vi "Main.vi"() -> ()   [LabVIEW 2019]
uses:
  <vilib>/NI/Current Value Table/Type Defs/File Format.ctl
  <vilib>/NI/Current Value Table/Type Defs/Single Tag.ctl
  <vilib>/NI/Current Value Table/Type Defs/Data Types.ctl
  <vilib>/NI/Current Value Table/Type Defs/Tag Grouping set.ctl
  QDMH support files/QDMH Poly VIs/QDMH POLY Enqueue String.vi
  <vilib>/NI/Current Value Table/Current Value Table.lvlib
panel:
  in  "Ordem de serviço 2":string
  in  "Temperatura 2":dbl
  in  "Temperatura 1":dbl
  in  "Ferramentas":string
  in  "Queue Name":string="Main-PoC"
  out "error out":errorcluster
  in  "error in (no error)":errorcluster
  out "Message Display":string
  in  "Cancel":bool
  in  "OK":bool
  in  "Ordem de serviço":string
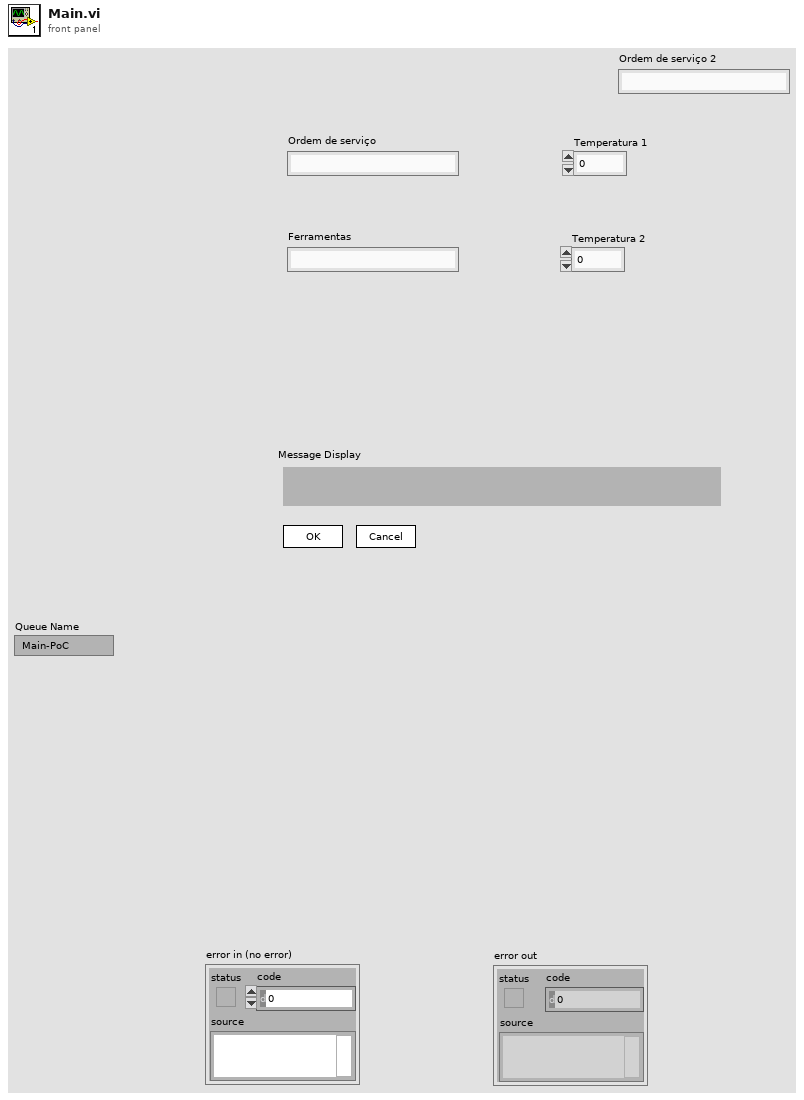
[diagram p1: front panel]
types:
  T1 = cluster{"Barcode to be sent":string, "Read code on next":bool, "New data?":bool, "SO code":cluster{"Current Barcode":string, "Ready to send?":bool, "New data to be polled?":bool}, "Tool code":cluster{"Current Barcode":string, "Ready to send?":bool, "New data to be polled?":bool}, "Polled Data to be sent":string}
  T2 = typedef "Current Value Table.lvlib/File Format.ctl" = cluster{"Tags":T3[], "Group Listings":T5[]}
  T3 = typedef "Current Value Table.lvlib/Single Tag.ctl" = cluster{"Data Type":T4, "Name":string, "Value":string, "Description":string}
  T4 = typedef "Current Value Table.lvlib/Data Types.ctl" = enum16{"Double", "Single", "I64", "I32", "I16", "I8", "U64", "U32", "U16", "U8", "String", "Boolean", "Array of U8", "Array of U16", "Array of U32", "Array of U64", "Array of I64", "Array of I32", "Array of I16", "Array of I8", "Array of Double", "Array of Single", "Array of Boolean", "Array of String"}
  T5 = typedef "Current Value Table.lvlib/Tag Grouping set.ctl" = cluster{"Group":string, "Tag Names":string[]}
  T6 = cluster{"SO Barcode":string, "Tool Barcode":string}
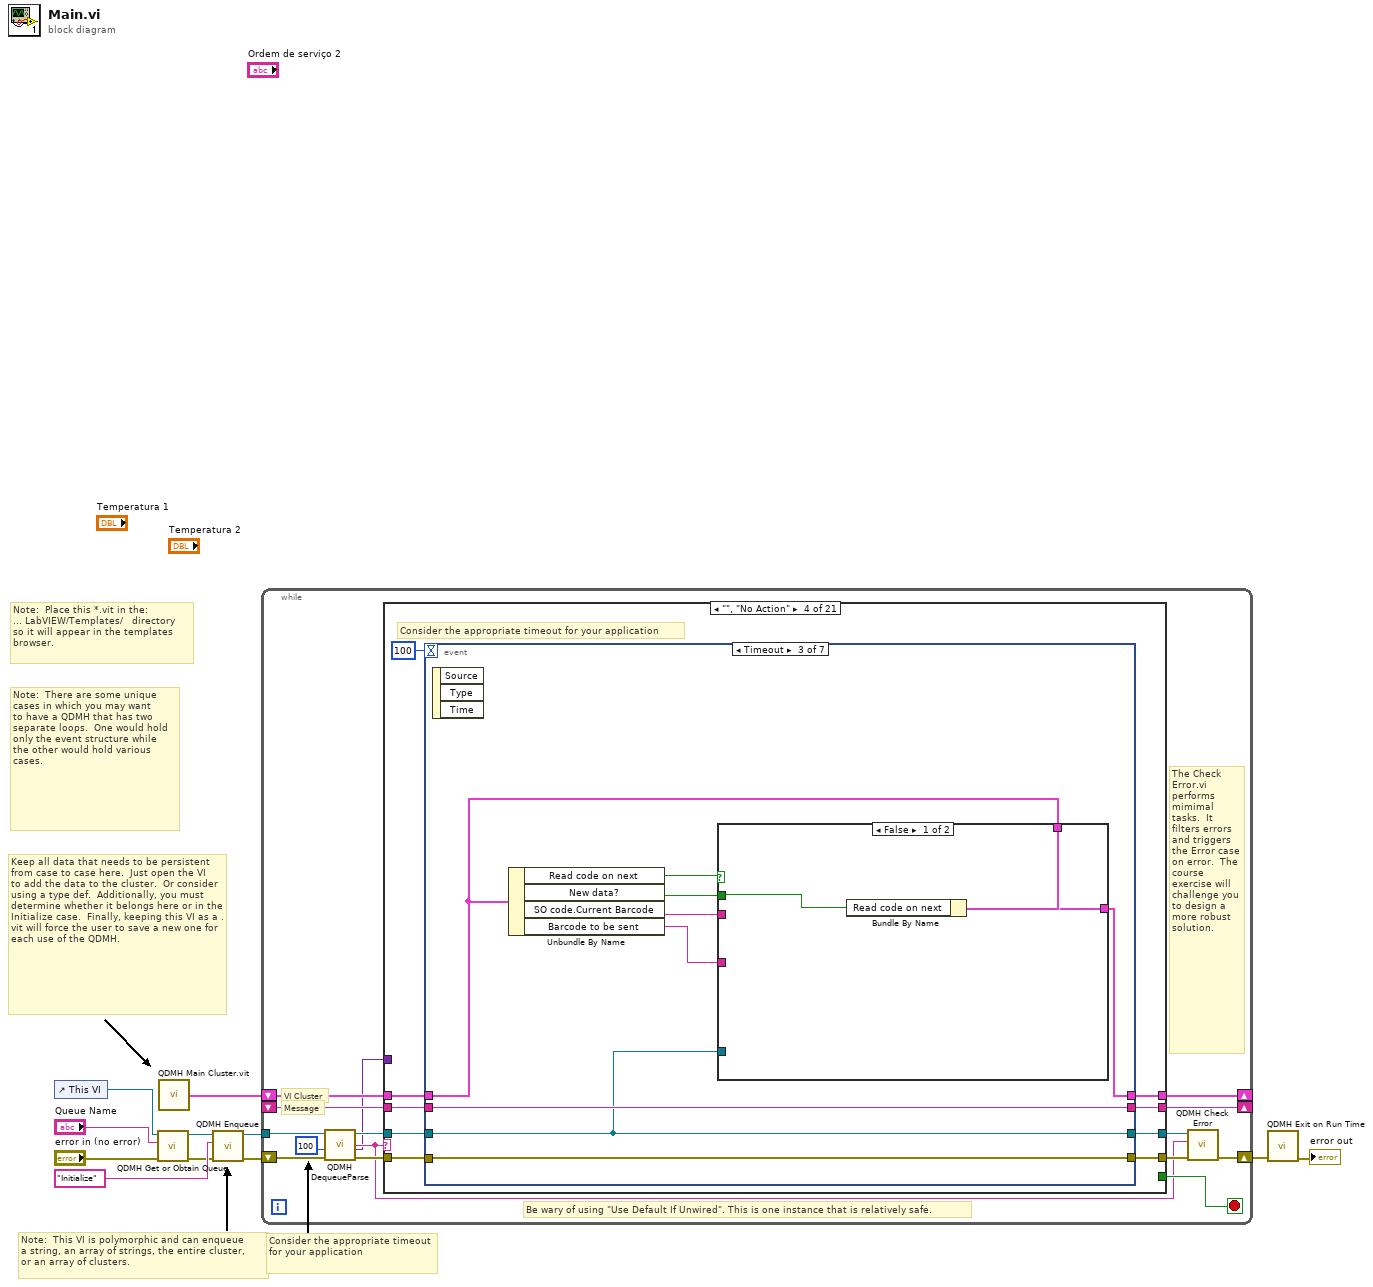
[diagram p0: block diagram]
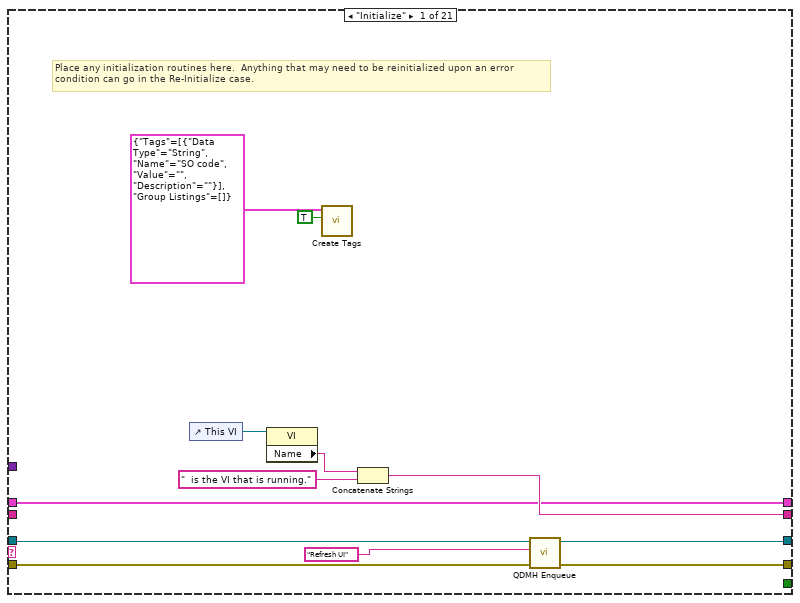
[diagram p2: hidden frame]
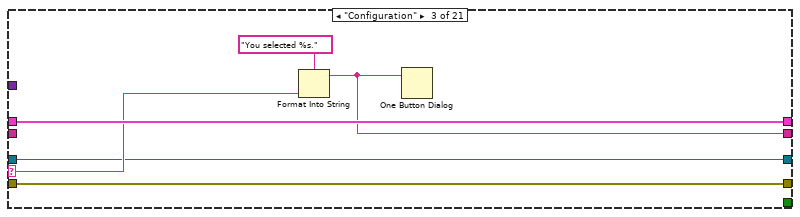
[diagram p4: hidden frame]
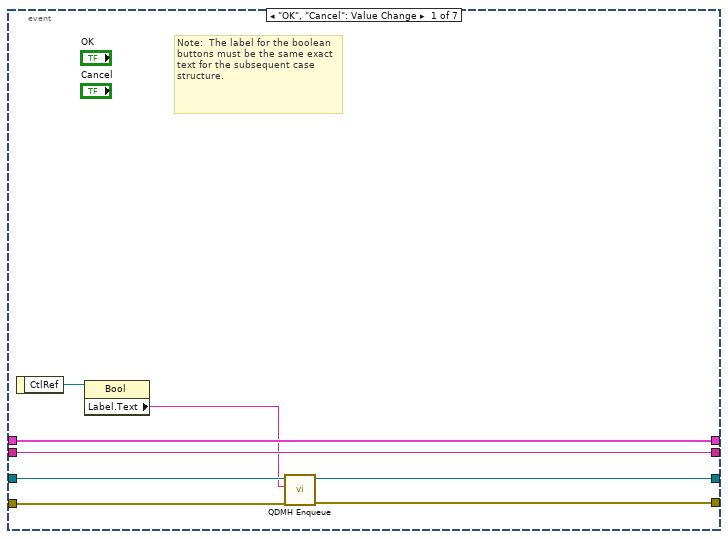
[diagram p5: hidden frame]
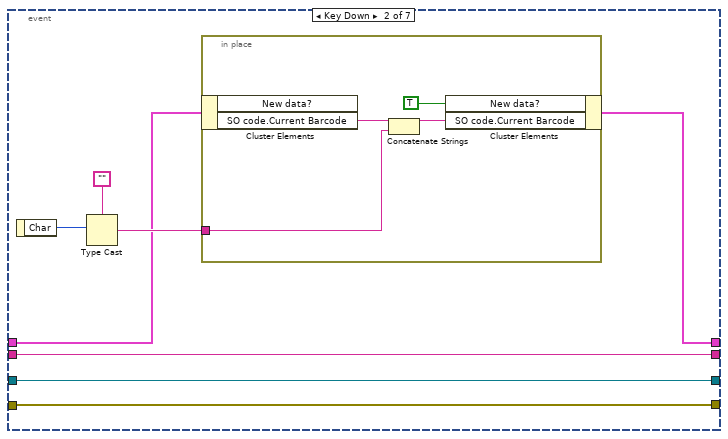
[diagram p6: hidden frame]
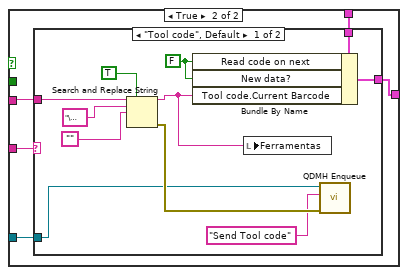
[diagram p7: hidden frame]
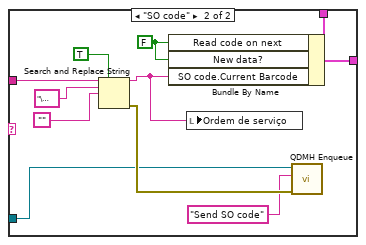
[diagram p8: hidden frame]
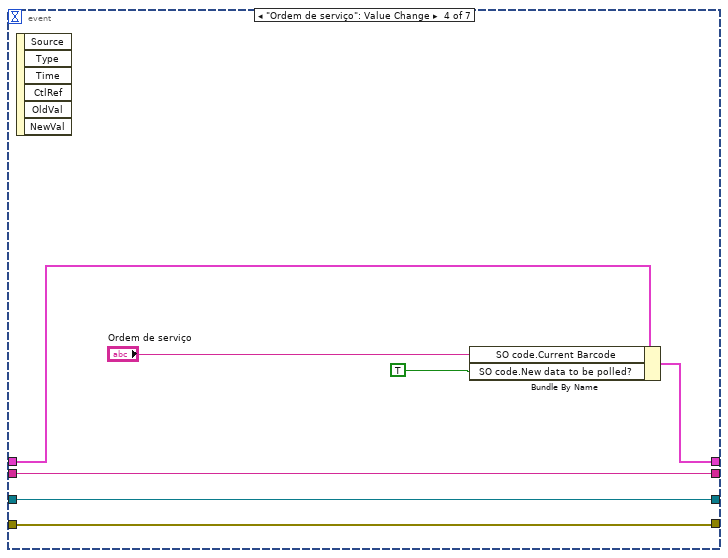
[diagram p9: hidden frame]
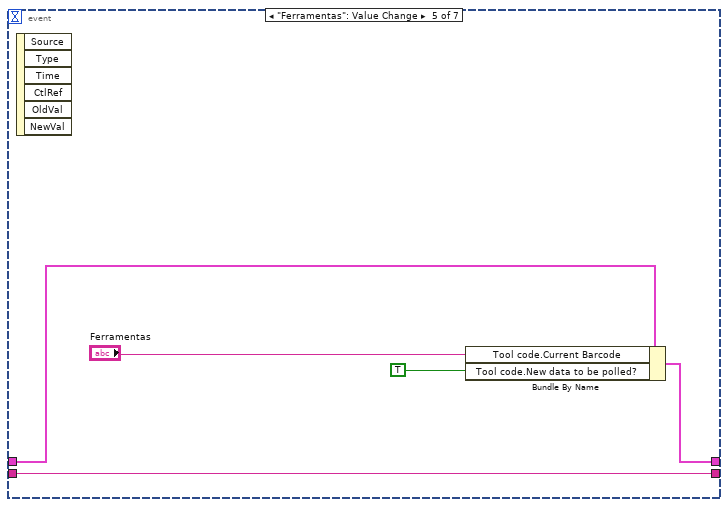
[diagram p10: hidden frame]
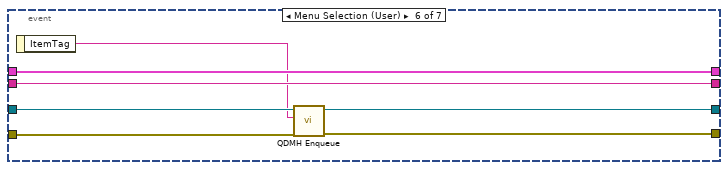
[diagram p11: hidden frame]
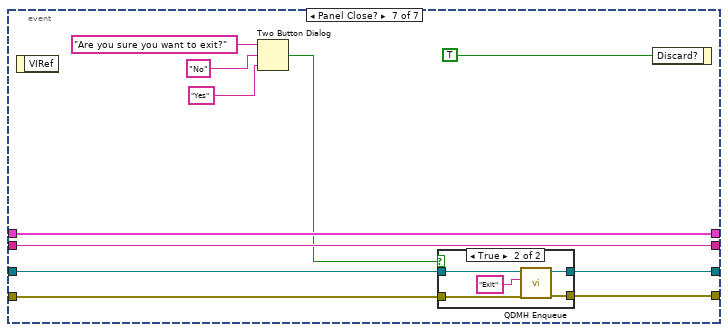
[diagram p12: hidden frame]
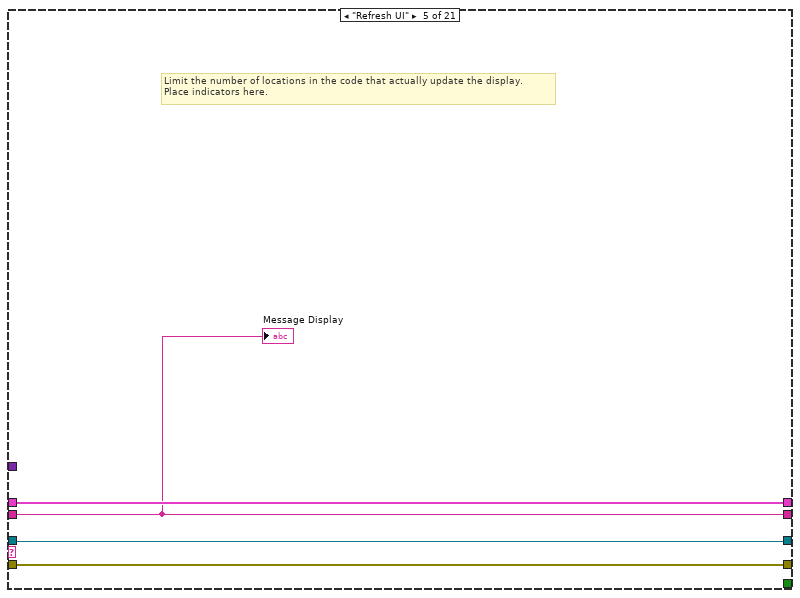
[diagram p14: hidden frame]
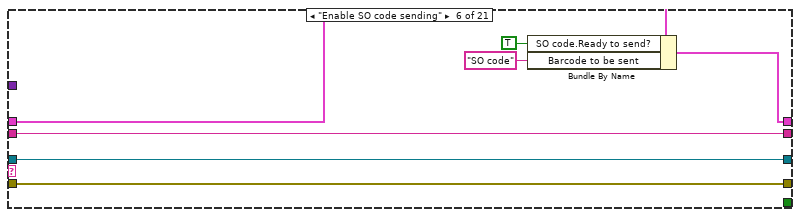
[diagram p15: hidden frame]
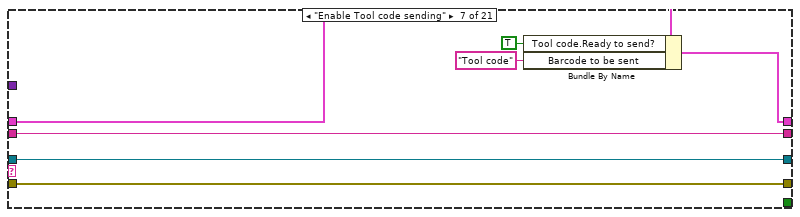
[diagram p16: hidden frame]
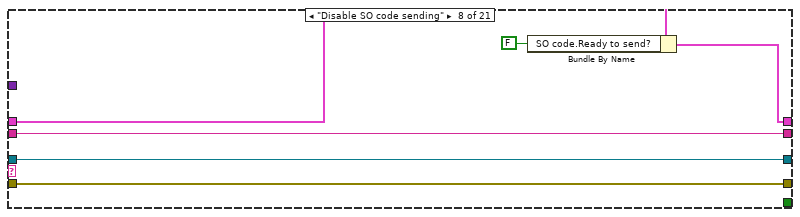
[diagram p17: hidden frame]
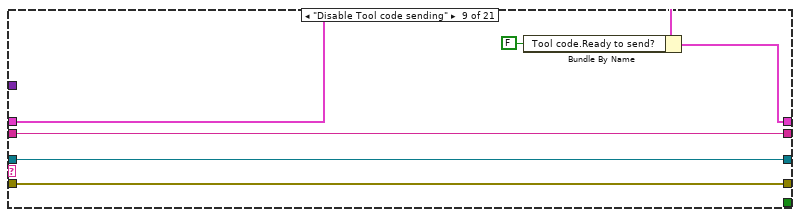
[diagram p18: hidden frame]
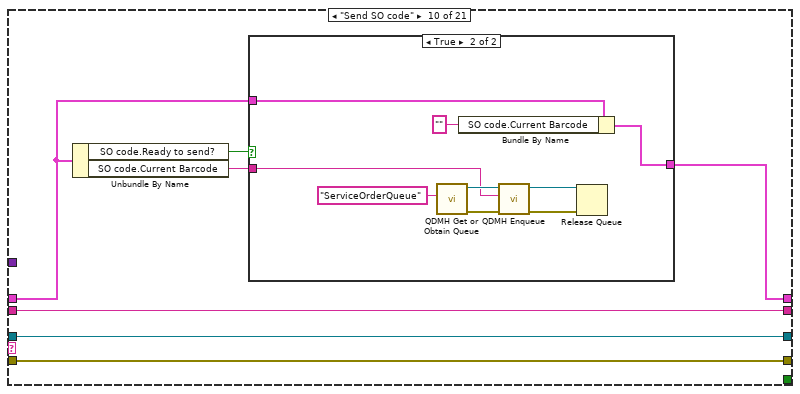
[diagram p19: hidden frame]
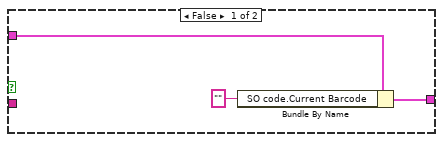
[diagram p20: hidden frame]
diagram:
  # "Consider the appropriate timeout for your application"
  # "Note:  There are some unique\ncases in which you may want\nto have a QDMH that has two\nseparate loops.  One would hold\nonly the event structure while\nthe other would hold various \ncases."
  # "Note:  Place this *.vit in the:\n... LabVIEW/Templates/   directory\nso it will appear in the templates\nbrowser."
  # "Note:  This VI is polymorphic and can enqueue\na string, an array of strings, the entire cluster,\nor an array of clusters."
  # "Keep all data that needs to be persistent\nfrom case to case here.  Just open the VI\nto add the data to the cluster.  Or consider \nusing a type def.  Additionally, you must determine whether it belongs here or in the Initialize case.  Finally, keeping this VI as a .vit will force the user to save a new one for each use of the QDMH."
  n1 = control-ref of="This VI"() -> (w3:refnum<vi>)
  n2 = call "QDMH Get or Obtain Queue.vi"("error in (no error)"="error in (no error)", "Queue Name"="Queue Name", "VI Refnum"=w3) -> ("error out"=w6:errorcluster, "queue out"=w7:refnum<queue>)  [unwired: 7 out]
  n3 = call "QDMH Main Cluster.vit"() -> ("Cluster"=w11:T1)
  n4 = call-poly "QDMH Enqueue.vi"("error in (no error)"=w6, "State"="Initialize" ("element"), "queue"=w7) -> ("error out"=w4:errorcluster, "queue out"=w5:refnum<queue>)  [unwired: 7 out]
  n5 = while {
    tunnel: w5 -> [w21]
    shift-left: w11 -> [w22]
    shift-right: [w23] -> _
    shift-left: _ -> [w24]
    shift-right: [w25] -> _
    shift-right: [w15] -> w2
    shift-left: w4 -> [w17]
    stop <- w26 stop-if-true
    # "Be wary of using \"Use Default If Unwired\". This is one instance that is relatively safe."
    # "VI Cluster"
    # "Message"
    # "The Check Error.vi performs mimimal tasks.  It filters errors and triggers the Error case on error.  The course exercise will challenge you to design a more robust solution."
    n6 = call "QDMH DequeueParse.vi"("error in (no error)"=w17, "Timeout"=100 ("ms timeout (-1)"), "queue"=w21) -> ("error out"=w18:errorcluster, "Variant Data"=w12:variant, "State"=w13:string, "queue out"=w19:refnum<queue>)  [unwired: 5 out]
    n7 = case shown="\"\", \"No Action\"" w13 {
      selector: w13 -> [_ _ w45 _ _ _ _ _ _ _ _ _ _ _ _ _ _ _ _ w310 _]
      tunnel: w19 -> [w36 w39 w44 w57 w155 w163 w170 w176 w182 w189 w208 w227 w262 w268 w275 w280 w290 w292 w304 w307 w319]
      tunnel: [_ _ _ _ _ _ _ _ _ _ _ _ _ _ _ _ _ _ _ _ TRUE] -> w26
      tunnel: [w34 w42 w46 w50 w156 w164 w171 w177 w183 w190 w209 w223 w263 w266 w276 w283 w289 w294 w306 w313 w321] -> w25
      tunnel: w24 -> [_ w42 _ w51 w156 w164 w171 w177 w183 w190 w209 w224 w263 w266 w276 w283 w289 w294 w306 w313 w321]
      tunnel: [w29 w41 w48 w52 w157 w161 w168 w174 w180 w184 w203 w222 w251 w265 w277 w282 w288 w293 w305 w312 w316] -> w23
      tunnel: w22 -> [w29 w41 w48 w53 w157 w160 w167 w173 w179 w185 w204 w222 w253 w265 w279 w282 w288 w293 w305 w312 w316]
      tunnel: w18 -> [w38 w40 w43 w56 w154 w162 w169 w175 w181 w188 w207 w231 w259 w267 w274 w281 w287 w291 _ w309 w318]
      tunnel: [w37 w40 w43 w55 w154 w162 w169 w175 w181 w188 w207 w228 w260 w267 w274 w281 w286 w291 w303 w309 w314] -> w16
      tunnel: [w30 w39 w44 w49 w155 w163 w170 w176 w182 w189 w208 w226 w261 w268 w275 w280 w284 w292 w302 w307 refnum<queue> refnum ("queue out")] -> w14
      tunnel: w12 -> [_ _ _ _ _ _ _ _ _ _ _ _ _ _ _ _ _ _ w300 _ _]
      frame "Initialize" {
        # "Place any initialization routines here.  Anything that may need to be reinitialized upon an error\ncondition can go in the Re-Initialize case."
        n8 = control-ref of="This VI"() -> (w33:refnum<vi>)
        n9 = property class="VI"(reference=w33) -> ("Name"=w32:string)  [unwired: 1 in, 2 out]
        n10 = call <vilib>:"Create Tags.vi"("Clear Table? (F)"=TRUE, "CVT Tags to Create"=T2 {"Tags"=[{"Data Type"=enum."String", "Name"="SO code", "Value"="", "Description"=""}], "Group Listings"=[]}) -> ()  [unwired: 9 in, 1 out]
        n11 = Concatenate Strings(w32, "  is the VI that is running." ("string")) -> (w34:string)
        n12 = call-poly "QDMH Enqueue.vi"("error in (no error)"=w38, "State"="Refresh UI" ("New State"), "queue"=w36) -> ("error out"=w37:errorcluster, "queue out"=w30:refnum<queue>)  [unwired: 7 out]
      }
      frame "Re-Initialize" {
        # "This case includes initialization functionality that may need to run again during the course of the VI"
      }
      frame "Configuration" {
        n13 = Format Into String(format string="You selected %s." ("Format String"), w45) -> (resulting string=w46:string)  [unwired: 2 in, 1 out]
        n14 = One Button Dialog(message=w46) -> ()  [unwired: 2 out]
      }
      frame "", "No Action" {
        # "Consider the appropriate timeout for your application"
        n15 = event shown="[2] Timeout" {
          selector: _ -> [_ _ _ _ _ _ _]
          dyn-events: _ -> [_ _ _ _ _ _ _]
          timeout: 100 -> [_ _ _ _ _ _ _]
          tunnel: w57 -> [w64 w68 w78 w118 _ w135 w141]
          tunnel: [w63 w67 w86 w117 _ w133 w138] -> w55
          tunnel: w56 -> [w62 w67 w86 w117 _ w134 w139]
          tunnel: w53 -> [w61 w69 w81 w122 w127 w132 w146]
          tunnel: [w61 w66 w80 w120 w126 w132 w146] -> w52
          tunnel: w51 -> [w60 w73 w85 w123 w128 w131 w145]
          tunnel: [w60 w73 w85 w123 w128 w131 w145] -> w50
          tunnel: [w58 w68 w78 w118 _ w129 w140] -> w49
          event "OK", "Cancel": Value Change {
            # "Note:  The label for the boolean buttons must be the same exact text for the subsequent case structure."
            n16 = event-data() -> ("CtlRef"=w65:refnum<vi>)  [unwired: 1 out]
            n17 = property class="Bool"(reference=w65) -> ("Label.Text"=w59:string)  [unwired: 1 in, 2 out]
            n18 = call-poly "QDMH Enqueue.vi"("error in (no error)"=w62, "State"=w59, "queue"=w64) -> ("error out"=w63:errorcluster, "queue out"=w58:refnum<queue>)  [unwired: 7 out]
          }
          event Key Down {
            n19 = event-data() -> ("Char"=w70:i16)  [unwired: 1 out]
            n20 = Type Cast(type="", x=w70) -> (*(type *) &x=w72:string)
            n21 = in-place {
              in-place-border: w72 -> [w76]
              n22 = in-place-cluster #1(w69) -> ("SO code.Current Barcode"=w77:string)  [unwired: 1 out]
              n23 = Concatenate Strings(w77, w76) -> (w75:string)
              n24 = in-place-cluster #1("New data?"=TRUE, "SO code.Current Barcode"=w75) -> (w66:T1)
            }
          }
          event Timeout {
            n25 = event-data() -> ()  [unwired: 4 out]
            n26 = Unbundle By Name(w81) -> ("Read code on next"=w83:bool, "New data?"=w84:bool, "SO code.Current Barcode"=w82:string, "Barcode to be sent"=w79:string)
            n27 = case shown="False" w83 {
              tunnel: w81 -> [w89 w92]
              tunnel: [w88 w93] -> w80
              tunnel: w84 -> [w87 _]
              tunnel: w82 -> [_ w94]
              tunnel: w79 -> [_ w90]
              tunnel: w78 -> [_ w91]
              frame False {
                n28 = Bundle By Name(cluster=w89, "Read code on next"=w87) -> (w88:T1)
              }
              frame True {
                n29 = case shown="\"Tool code\", Default" w90 {
                  tunnel: w94 -> [w100 w115]
                  tunnel: [w97 w112] -> w93
                  tunnel: w92 -> [w96 w110]
                  tunnel: w91 -> [w99 w108]
                  frame "Tool code", Default {
                    w104 = FALSE ("QR codes.Read code on next")
                    n30 = Search and Replace String(replace all?=TRUE ("replace all? (F)"), input string=w100, search string="\u0000", replace string="") -> (result string=w95:string, error out=w105:errorcluster)  [unwired: 4 in, 2 out]
                    n31 = Bundle By Name(cluster=w96, "Read code on next"=w104, "New data?"=w104, "Tool code.Current Barcode"=w95) -> (w97:T1)
                    n32 = local write "Ferramentas"(w95) -> ()
                    n33 = call-poly "QDMH Enqueue.vi"("error in (no error)"=w105, "State"="Send Tool code", "queue"=w99) -> ()  [unwired: 9 out]
                  }
                  frame "SO code" {
                    w111 = FALSE ("QR codes.Read code on next")
                    n34 = Search and Replace String(replace all?=TRUE ("replace all? (F)"), input string=w115, search string="\u0000", replace string="") -> (result string=w106:string, error out=w109:errorcluster)  [unwired: 4 in, 2 out]
                    n35 = Bundle By Name(cluster=w110, "Read code on next"=w111, "New data?"=w111, "SO code.Current Barcode"=w106) -> (w112:T1)
                    n36 = local write "Ordem de serviço"(w106) -> ()
                    n37 = call-poly "QDMH Enqueue.vi"("error in (no error)"=w109, "State"="Send SO code", "queue"=w108) -> ()  [unwired: 9 out]
                  }
                }
              }
            }
          }
          event "Ordem de serviço": Value Change {
            n38 = event-data() -> ()  [unwired: 7 out]
            n39 = Bundle By Name(cluster=w122, "SO code.Current Barcode"="Ordem de serviço", "SO code.New data to be polled?"=TRUE ("SO code.Ready to be polled?")) -> (w120:T1)
          }
          event "Ferramentas": Value Change {
            n40 = event-data() -> ()  [unwired: 7 out]
            n41 = Bundle By Name(cluster=w127, "Tool code.Current Barcode"="Ferramentas", "Tool code.New data to be polled?"=TRUE ("SO code.Ready to be polled?")) -> (w126:T1)
          }
          event Menu Selection (User) {
            n42 = event-data() -> ("ItemTag"=w130:string)  [unwired: 1 out]
            n43 = call-poly "QDMH Enqueue.vi"("error in (no error)"=w134, "State"=w130, "queue"=w135) -> ("error out"=w133:errorcluster, "queue out"=w129:refnum<queue>)  [unwired: 7 out]
          }
          event Panel Close? {
            n44 = event-data() -> ()  [unwired: 2 out]
            n45 = Two Button Dialog(message="Are you sure you want to exit?", 1:"Yes" ("F button name (\"Cancel\")"), 2:"No" ("T button name (\"OK\")")) -> (T button?=w137:bool)
            n46 = case shown="True" w137 {
              tunnel: w141 -> [w148 w153]
              tunnel: [w148 w152] -> w140
              tunnel: w139 -> [w147 w151]
              tunnel: [w147 w150] -> w138
              frame False {
              }
              frame True {
                n47 = call-poly "QDMH Enqueue.vi"("error in (no error)"=w151, "State"="Exit", "queue"=w153) -> ("error out"=w150:errorcluster, "queue out"=w152:refnum<queue>)  [unwired: 7 out]
              }
            }
            n48 = event-data("Discard?"=TRUE) -> ()  [unwired: 1 in, 1 out]
          }
        }
      }
      frame "Refresh UI" {
        # "Limit the number of locations in the code that actually update the display.\nPlace indicators here."
        "Message Display" <- w156
      }
      frame "Enable SO code sending" {
        n49 = Bundle By Name(cluster=w160, "SO code.Ready to send?"=TRUE ("QR codes.Ready to send?"), "Barcode to be sent"="SO code") -> (w161:T1)
      }
      frame "Enable Tool code sending" {
        n50 = Bundle By Name(cluster=w167, "Tool code.Ready to send?"=TRUE ("QR codes.Ready to send?"), "Barcode to be sent"="Tool code") -> (w168:T1)
      }
      frame "Disable SO code sending" {
        n51 = Bundle By Name(cluster=w173, "SO code.Ready to send?"=FALSE ("QR codes.Ready to send?")) -> (w174:T1)
      }
      frame "Disable Tool code sending" {
        n52 = Bundle By Name(cluster=w179, "Tool code.Ready to send?"=FALSE ("QR codes.Ready to send?")) -> (w180:T1)
      }
      frame "Send SO code" {
        n53 = Unbundle By Name(w185) -> ("SO code.Ready to send?"=w187:bool, "SO code.Current Barcode"=w186:string)
        n54 = case shown="True" w187 {
          tunnel: w186 -> [_ w197]
          tunnel: w185 -> [w193 w196]
          tunnel: [w191 w195] -> w184
          frame False {
            n55 = Bundle By Name(cluster=w193, "SO code.Current Barcode"="" ("QR codes.Current QR code")) -> (w191:T1)
          }
          frame True {
            n56 = call "QDMH Get or Obtain Queue.vi"("Queue Name"="ServiceOrderQueue") -> ("error out"=w200:errorcluster, "queue out"=w201:refnum<queue>)  [unwired: 2 in, 7 out]
            n57 = Bundle By Name(cluster=w196, "SO code.Current Barcode"="" ("QR codes.Current QR code")) -> (w195:T1)
            n58 = call-poly "QDMH Enqueue.vi"("error in (no error)"=w200, "State"=w197, "queue"=w201) -> ("error out"=w198:errorcluster, "queue out"=w199:refnum<queue>)  [unwired: 7 out]
            n59 = Release Queue(queue=w199, error in (no error)=w198) -> ()  [unwired: 1 in, 3 out]
          }
        }
      }
      frame "Send Tool code" {
        n60 = Unbundle By Name(w204) -> ("Tool code.Ready to send?"=w206:bool, "SO code.Current Barcode"=w205:string)
        n61 = case shown="True" w206 {
          tunnel: w205 -> [_ w216]
          tunnel: w204 -> [w212 w215]
          tunnel: [w210 w214] -> w203
          frame False {
            n62 = Bundle By Name(cluster=w212, "SO code.Current Barcode"="" ("QR codes.Current QR code")) -> (w210:T1)
          }
          frame True {
            n63 = call "QDMH Get or Obtain Queue.vi"("Queue Name"="ToolQueue") -> ("error out"=w219:errorcluster, "queue out"=w220:refnum<queue>)  [unwired: 2 in, 7 out]
            n64 = Bundle By Name(cluster=w215, "SO code.Current Barcode"="" ("QR codes.Current QR code")) -> (w214:T1)
            n65 = call-poly "QDMH Enqueue.vi"("error in (no error)"=w219, "State"=w216, "queue"=w220) -> ("error out"=w217:errorcluster, "queue out"=w218:refnum<queue>)  [unwired: 7 out]
            n66 = Release Queue(queue=w218, error in (no error)=w217) -> ()  [unwired: 1 in, 3 out]
          }
        }
      }
      frame "New data to poll?" {
        n67 = Unbundle By Name(w222) -> ("SO code.New data to be polled?"=w230:bool, "Tool code.New data to be polled?"=w229:bool)
        n68 = Or(x=w230, y=w229) -> (x .or. y?=w225:bool)
        n69 = case shown="True" w225 {
          tunnel: w231 -> [w239 w250]
          tunnel: [w239 w245] -> w228
          tunnel: w227 -> [w240 w248]
          tunnel: [w240 w243] -> w226
          tunnel: w224 -> [w241 w247]
          tunnel: [w241 w247] -> w223
          frame False {
            n70 = Flatten To JSON(anything=T6 {"SO Barcode"="", "Tool Barcode"=""}) -> (JSON string=w232:string)  [unwired: 2 in, 1 out]
            n71 = call "QDMH Get or Obtain Queue.vi"("Queue Name"="PollDataQueue") -> ("error out"=w236:errorcluster, "queue out"=w237:refnum<queue>)  [unwired: 2 in, 7 out]
            n72 = call-poly "QDMH Enqueue.vi"("error in (no error)"=w236, "State"=w232, "queue"=w237) -> ("error out"=w234:errorcluster, "queue out"=w235:refnum<queue>)  [unwired: 7 out]
            n73 = Release Queue(queue=w235, error in (no error)=w234) -> ()  [unwired: 1 in, 3 out]
          }
          frame True {
            n74 = call-poly "QDMH Enqueue.vi"("error in (no error)"=w250, "State"="Format Polled Data", "queue"=w248) -> ("error out"=w249:errorcluster, "queue out"=w244:refnum<queue>)  [unwired: 7 in]
            n75 = call-poly "QDMH Enqueue.vi"("error in (no error)"=w249, "State"="Send Polled Data", "queue"=w244) -> ("error out"=w245:errorcluster, "queue out"=w243:refnum<queue>)  [unwired: 7 in]
          }
        }
      }
      frame "Format Polled Data" {
        n76 = Unbundle By Name(w253) -> ("SO code.Current Barcode"=w257:string, "Tool code.Current Barcode"=w256:string)
        n77 = Bundle By Name(cluster=T6 {"SO Barcode"="", "Tool Barcode"=""}, "SO Barcode"=w257, "Tool Barcode"=w256) -> (w255:T6)
        n78 = Flatten To JSON(anything=w255) -> (JSON string=w252:string)  [unwired: 2 in, 1 out]
        n79 = Bundle By Name(cluster=w253, "Polled Data to be sent"=w252) -> (w251:T1)
        n80 = call-poly "QDMH Enqueue.vi"("error in (no error)"=w259, "State"="Send Polled Data", "queue"=w262) -> ("error out"=w260:errorcluster, "queue out"=w261:refnum<queue>)  [unwired: 7 out]
      }
      frame "Send Polled Data" {
        n81 = Unbundle By Name(w265) -> ("Polled Data to be sent"=w264:string)
        n82 = call "QDMH Get or Obtain Queue.vi"("Queue Name"="PollDataQueue") -> ("error out"=w271:errorcluster, "queue out"=w272:refnum<queue>)  [unwired: 2 in, 7 out]
        n83 = call-poly "QDMH Enqueue.vi"("error in (no error)"=w271, "State"=w264, "queue"=w272) -> ("error out"=w269:errorcluster, "queue out"=w270:refnum<queue>)  [unwired: 7 out]
        n84 = Release Queue(queue=w270, error in (no error)=w269) -> ()  [unwired: 1 in, 3 out]
      }
      frame "Clear polling data" {
        w278 = FALSE ("SO code.New data to be polled?")
        n85 = Bundle By Name(cluster=w279, "SO code.New data to be polled?"=w278, "Tool code.New data to be polled?"=w278) -> (w277:T1)
      }
      frame "<duplicate me for new states >" {
        # "Duplicate this state for any additional states that you add."
      }
      frame "OK" {
        n86 = call-poly "QDMH Enqueue.vi"("error in (no error)"=w287, "State"="Exit" ("New State"), "queue"=w290) -> ("error out"=w286:errorcluster, "queue out"=w284:refnum<queue>)  [unwired: 7 out]
      }
      frame "Cancel" {
      }
      frame "Error" {
        # "This codes simply displays an error dialog that will allow the user\nto continue code execution or Exit.  More error correction code\ncould be included.  This will be explored in the error system exercise."
        n87 = Variant To Data(type=cluster{"Case":string, "error":errorcluster} {"Case"="", "error"={"status"=FALSE, "code"=0, "source"=""}} ("QDSM Element"), Variant=w300) -> (data=w299:cluster{"Case":string, "error":errorcluster})  [unwired: 1 in, 1 out]
        n88 = Unbundle By Name(w299) -> ("Case"=w298:string, "error"=w297:errorcluster)
        n89 = call "QDMH Error Dialog.vi"("error"=w297, "Case Error Occured"=w298) -> ("error out (no error)"=w295:errorcluster, "Case to Execute"=w296:string)  [unwired: 8 out]
        n90 = call-poly "QDMH Enqueue.vi"("error in (no error)"=w295, "State"=w296, "queue"=w304) -> ("error out"=w303:errorcluster, "queue out"=w302:refnum<queue>)  [unwired: 7 out]
      }
      frame "Developer Error", Default {
        # "Many eschew the use of string based state machines because of the propensity for\ntypos, prefering instead to use enums.  This case eliminates that concern.\nPerhaps modify to exit the VI."
        n91 = Format Into String(format string="Developer Error: The requested state \"%s\" does not exist." ("message"), w310) -> (resulting string=w308:string)  [unwired: 2 in, 1 out]
        n92 = One Button Dialog(message=w308) -> ()  [unwired: 2 out]
      }
      frame "Exit" {
        # "Note:  The release queue function has the force destroy option set to true."
        # "Place any critical clean up routines here."
        n93 = Release Queue(queue=w319, force destroy? (F)=TRUE, error in (no error)=w318) -> (error out=w314:errorcluster)  [unwired: 2 out]
        n94 = local write "Message Display"("") -> ()
      }
    }
    n95 = call "QDMH Check Error.vi"("error in (no error)"=w16, "Case"=w13, "queue"=w14) -> ("error out"=w15:errorcluster)  [unwired: 1 in, 7 out]
  }
  n96 = call "QDMH Exit on Run Time.vi"("error in (no error)"=w2) -> ("error out"=→"error out":errorcluster)  [unwired: 10 in]
